vi "[FGV]ProcessDataEntry.vi"(7 "ProcessDataEntry_Action":T3, 8 "Error In":errorcluster, 9 "OldAllProcessSetting In":T1[](array[typedef]), 10 "Prcocess Step":i32, 11 "AllProcessSetting In":T1[](array[typedef])) -> (0 "Error Out":errorcluster, 1 "OldAllProcessSetting Out":T1[](array[typedef]), 2 "ProcessSetting Out":T1={"Enum_PreProcess"=enum."CamAttributes", "Parameter"=""}, 3 "AllProcessSettingOut":T1[](array[typedef]))   [LabVIEW 2019]
uses:
  Controls/Process_Setting.ctl
  Ctrl/VisionProcessName.ctl
  Controls/ProcessDataEntry_Action.ctl
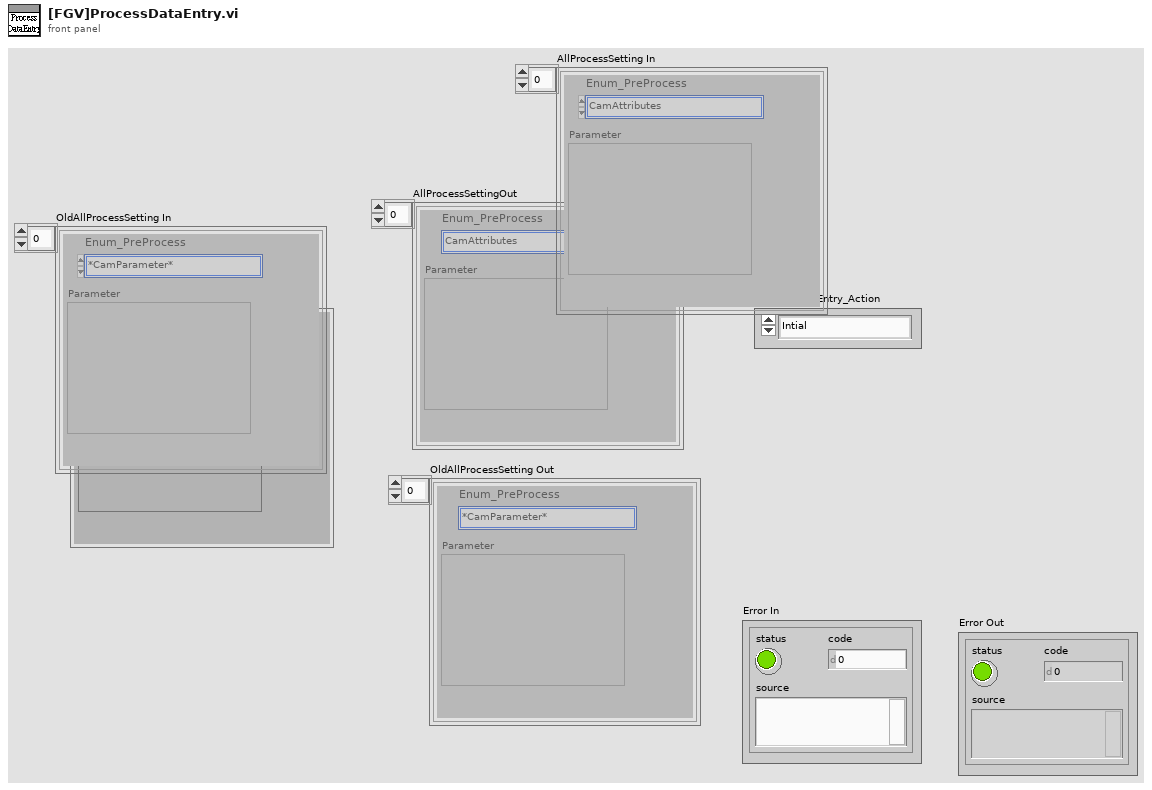
[diagram p1: front panel]
types:
  T1 = typedef "Process_Setting.ctl" = cluster{"Enum_PreProcess":T2, "Parameter":string}
  T2 = typedef "VisionProcessName.ctl" = enum16{"*CamParameter*", "CamAttributes", "*Preprocess*", "CG_Brightness", "C_Plane Extraction", "C_Threshold", "G_Lookup Table", "G_Threshold"}
  T3 = typedef "ProcessDataEntry_Action.ctl" = enum16{"Intial", "UpdateSteps", "ReallAllSteps", "ReadStep"}
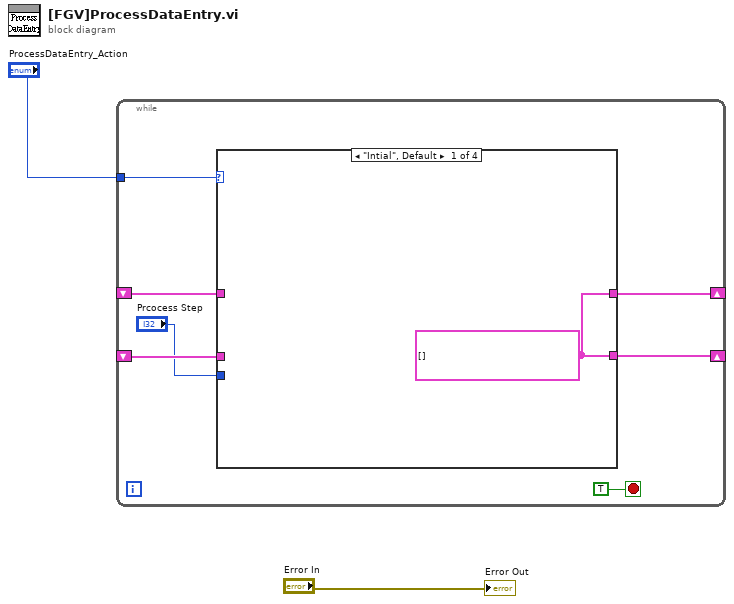
[diagram p0: block diagram]
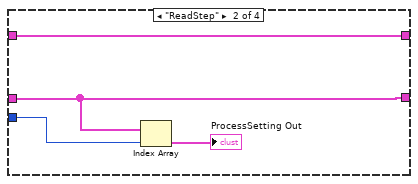
[diagram p2: hidden frame]
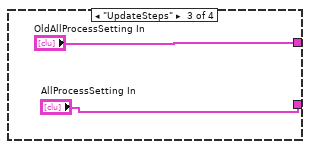
[diagram p3: hidden frame]
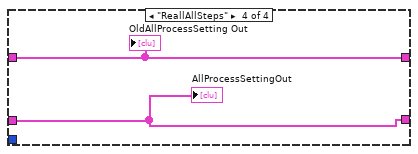
[diagram p4: hidden frame]
diagram:
  n1 = while {
    shift-right: [w7] -> _
    shift-left: _ -> [w6]
    tunnel: "ProcessDataEntry_Action" -> [w8]
    shift-right: [w4] -> _
    shift-left: _ -> [w3]
    stop <- TRUE stop-if-true
    n2 = case shown="\"Intial\", Default" w8 {
      tunnel: [w10 w13 "AllProcessSetting In" w18] -> w7
      tunnel: w6 -> [_ w13 _ w18]
      tunnel: "Prcocess Step" -> [_ w14 _ _]
      tunnel: [w10 w11 "OldAllProcessSetting In" w17] -> w4
      tunnel: w3 -> [_ w11 _ w17]
      frame "Intial", Default {
        w10 = T1[] [] ("ProcessSettingIn")
      }
      frame "ReadStep" {
        n3 = Index Array(array=w13, index=w14) -> (element=→"ProcessSetting Out":T1)
      }
      frame "UpdateSteps" {
      }
      frame "ReallAllSteps" {
        "AllProcessSettingOut" <- w18
        "OldAllProcessSetting Out" <- w17
      }
    }
  }
  "Error Out" <- "Error In"
